vi "XOR Encryption - (4) Key Rotation (2017 Channel Wire).vi"() -> ()   [LabVIEW 2016]
uses:
  <extravilib>/ChannelInstances/Stream-str/Write With Abort.vi
  <extravilib>/ChannelInstances/Stream-str/Read With Abort.vi
  <extravilib>/ChannelInstances/Stream-str/Endpoint.vi
  <extravilib>/ChannelInstances/Stream-str/EndpointRead.vi
  <extravilib>/ChannelInstances/Stream-str/Instantiate.vi
  <extravilib>/ChannelInstances/Stream-str/)Channel.vi
  <resource>/ChannelSupport/_ChannelSupport/WaitIfNeeded.vi
  <extravilib>/ChannelInstances/Stream-str.lvlib
panel:
  out "key out":string
  out "Rx Key":string
  out "data out 2":string
  out "Initial Key":string
  out "Data Out":string[](array[string])
  in  "Data In":string[](array[string])=["Hello", "LabVIEW", "World"]
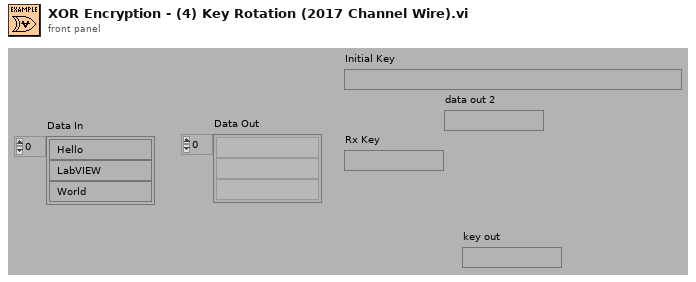
[diagram p1: front panel]
types:
  T1 = typedef "Stream-str.lvlib/)Channel.ctl" = refnum<queue>
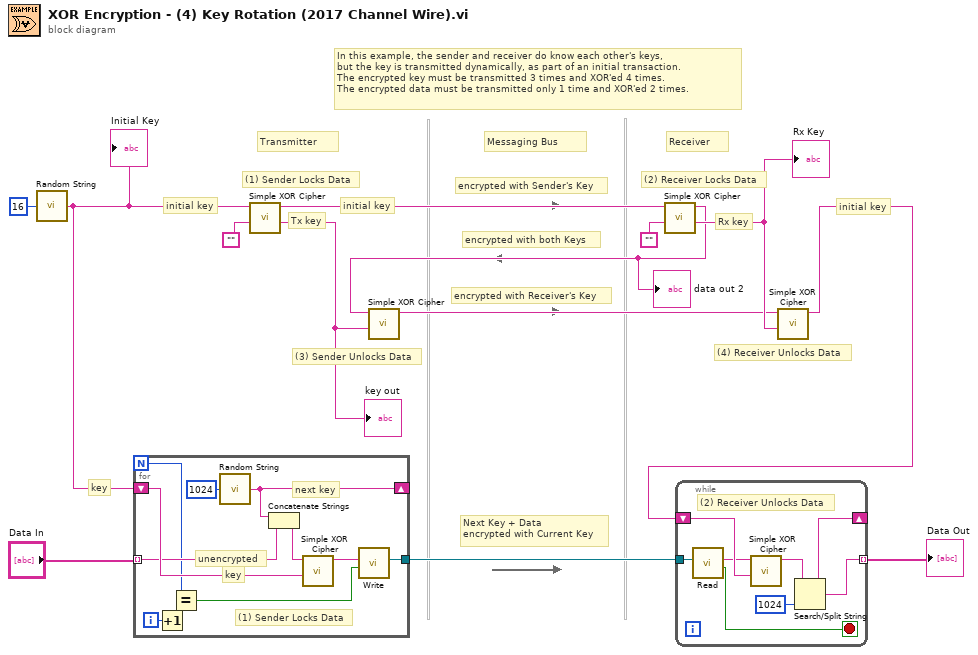
[diagram p0: block diagram]
diagram:
  # "key"
  # "initial key"
  # "initial key"
  # "Next Key + Data\nencrypted with Current Key"
  # "Messaging Bus"
  # "Receiver"
  # "Transmitter"
  # "initial key"
  # "Rx key"
  # "Tx key"
  # "In this example, the sender and receiver do know each other's keys,\nbut the key is transmitted dynamically, as part of an initial transaction.\nThe encrypted key must be transmitted 3 times and XOR'ed 4 times.\nThe encrypted data must be transmitted only 1 time and XOR'ed 2 times."
  # "encrypted with Receiver's Key"
  # "encrypted with Sender's Key"
  # "encrypted with both Keys"
  # "(4) Receiver Unlocks Data"
  # "(3) Sender Unlocks Data"
  # "(2) Receiver Locks Data"
  # "(1) Sender Locks Data"
  n1 = call "Random String.vi"("length"=16) -> ("random data"=w9:string)  [unwired: 4 in]
  "Initial Key" <- w9
  n2 = for {
    N -> [w16]
    shift-right: [w21] -> _
    shift-left: w9 -> [w24]
    tunnel: "Data In" -> [w20] mode=indexing
    tunnel: [w18] -> w5
    i -> [w17]
    # "key"
    # "next key"
    # "unencrypted"
    # "(1) Sender Locks Data"
    n3 = Increment(x=w17) -> (x+1=w15:i32)
    n4 = Equal?(x=w16, y=w15) -> (x = y?=w14:bool)
    n5 = call "Random String.vi"("length"=1024) -> ("random data"=w21:string)  [unwired: 4 in]
    n6 = Concatenate Strings(w21, w20) -> (w22:string)
    n7 = call "Simple XOR Cipher.vi"("key (\"\": random)"=w24, "data in"=w22) -> ("data out"=w19:string)  [unwired: 8 in, 1 out]
    n8 = call <extravilib>:"Write.vi"("last element? (F)"=w14, "element"=w19) -> ("channel"=w18:T1)  [unwired: 7 in, 2 out]
  }
  n9 = call "Simple XOR Cipher.vi"("key (\"\": random)"="", "data in"=w9) -> ("key out"=w13:string, "data out"=w1:string)  [unwired: 8 in]
  "key out" <- w13
  n10 = call "Simple XOR Cipher.vi"("key (\"\": random)"="", "data in"=w1) -> ("key out"=w4:string, "data out"=w3:string)  [unwired: 8 in]
  "data out 2" <- w3
  "Rx Key" <- w4
  n11 = call "Simple XOR Cipher.vi"("key (\"\": random)"=w13, "data in"=w3) -> ("data out"=w2:string)  [unwired: 8 in, 1 out]
  n12 = call "Simple XOR Cipher.vi"("key (\"\": random)"=w4, "data in"=w2) -> ("data out"=w8:string)  [unwired: 8 in, 1 out]
  n13 = while {
    tunnel: [w28] -> w6 mode=indexing
    tunnel: w5 -> [w27]
    shift-right: [w29] -> _
    shift-left: w8 -> [w32]
    stop <- w26 stop-if-true
    # "(2) Receiver Unlocks Data"
    n14 = call <extravilib>:"Read.vi"("channel"=w27) -> ("last element?"=w26:bool, "element"=w25:string)  [unwired: 6 in, 3 out]
    n15 = call "Simple XOR Cipher.vi"("key (\"\": random)"=w32, "data in"=w25) -> ("data out"=w30:string)  [unwired: 8 in, 1 out]
    n16 = Search/Split String(string=w30, offset (0)=1024) -> (substring before match=w29:string, match + rest of string=w28:string)  [unwired: 1 in, 1 out]
  }
  "Data Out" <- w6
